vi "SystemTimeStamptoCVT.vi"(8 "error in (no error)":errorcluster, 11 "BaseDriver in":refnum<class "BaseDriver.lvclass">) -> (0 "error out":errorcluster, 3 "BaseDriver out":refnum<class "BaseDriver.lvclass">)   [LabVIEW 2020, in "BaseDriver.lvclass"]
doc: "This VI does 2 things - \n\n1. It updates a variable called system timestamp in the CVT\n2. If the scan is OFF and save is ON, the timestamp information is used to put into the filename.\n\nNOTE - If the custom timestamp is updated anywhere in the acquire case, that information is used for\nlabelling, if not then the systemtimestamp is used for labelling"
uses:
  BaseDriver.lvclass
  BaseDriver.lvclass/BaseDriver.ctl
panel:
  out "SysTmestamp":dbl format="%.3f"
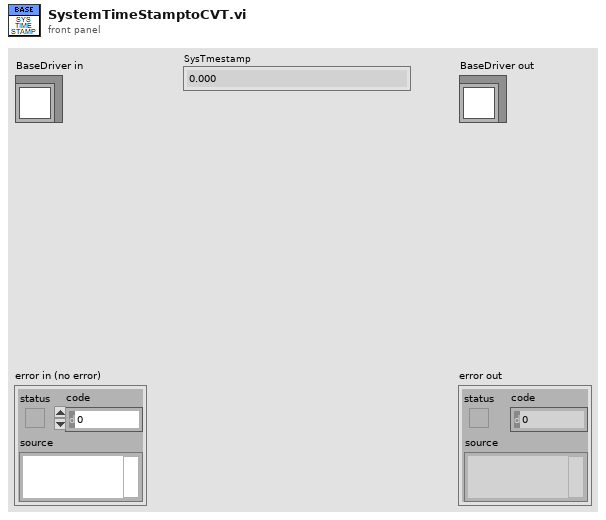
[diagram p1: front panel]
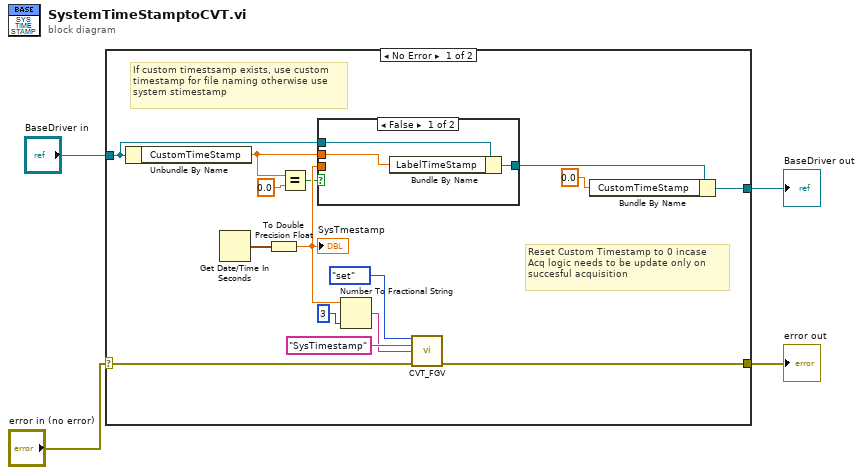
[diagram p0: block diagram]
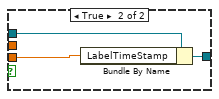
[diagram p2: hidden frame]
diagram:
  n1 = case shown="No Error" "error in (no error)" {
    selector: "error in (no error)" -> [w16 w27]
    tunnel: [w15 w27] -> w4
    tunnel: [w6 w26] -> w2
    tunnel: "BaseDriver in" -> [w9 w26]
    frame No Error {
      # "Reset Custom Timestamp to 0 incase\nAcq logic needs to be update only on \nsuccesful acquisition"
      # "If custom timestsamp exists, use custom\ntimestamp for file naming otherwise use\nsystem stimestamp"
      n2 = Unbundle By Name(w9) -> ("CustomTimeStamp"=w8:dbl)
      n3 = Get Date/Time In Seconds() -> (seconds since 1Jan1904=w19:timestamp)
      n4 = To Double Precision Float(number=w19) -> (double precision float=w12:dbl)
      "SysTmestamp" <- w12
      n5 = Equal?(x=w8, y=0.0) -> (x = y?=w10:bool)
      n6 = case shown="False" w10 {
        tunnel: w9 -> [w21 w25]
        tunnel: w12 -> [_ w24]
        tunnel: [w22 w23] -> w7
        tunnel: w8 -> [w20 _]
        frame False {
          n7 = Bundle By Name(cluster=w21, "LabelTimeStamp"=w20) -> (w22:refnum<class "BaseDriver.lvclass">)
        }
        frame True {
          n8 = Bundle By Name(cluster=w25, "LabelTimeStamp"=w24) -> (w23:refnum<class "BaseDriver.lvclass">)
        }
      }
      n9 = Number To Fractional String(number=w12, precision (6)=i16 3) -> (F-format string=w14:string)  [unwired: 2 in]
      n10 = call "CVT_FGV.vi"("command"=enum16{"set", "get", "reset", "get all"}."set", "variable"="SysTimestamp", "value in"=w14, "error in"=w16) -> ("error out"=w15:errorcluster)  [unwired: 9 in, 2 out]
      n11 = Bundle By Name(cluster=w7, "CustomTimeStamp"=0.0 ("y")) -> (w6:refnum<class "BaseDriver.lvclass">)
    }
    frame Error {
    }
  }
  "error out" <- w4
  "BaseDriver out" <- w2
